vi "Digital Write Square Wave.vi"(7 "Duration (ms)":u32, 8 "Error In":errorcluster, 9 "Frequency":u16, 10 "DO Channel":u8, 11 "LINX Device Config":T1) -> (0 "Error Out":errorcluster, 3 "LINX Device Config":T1)   [LabVIEW 2013, in "LVH-LINX.lvlib" / "Device.lvlib"]
uses:
  <vilib>/LabVIEW Hacker/LINX/Private/Device/Device.lvlib
  <vilib>/LabVIEW Hacker/LINX/Private/Device/Type Defs/LINX Device Config.ctl
  <vilib>/LabVIEW Hacker/LINX/Private/Type Defs/Interface.ctl
  <vilib>/LabVIEW Hacker/LINX/Private/Device/Type Defs/TCP Config.ctl
  <vilib>/LabVIEW Hacker/LINX/Private/Type Defs/Device Family.ctl
  <vilib>/LabVIEW Hacker/LINX/Private/Type Defs/Error Type.ctl
  <vilib>/LabVIEW Hacker/LINX/LVH-LINX.lvlib
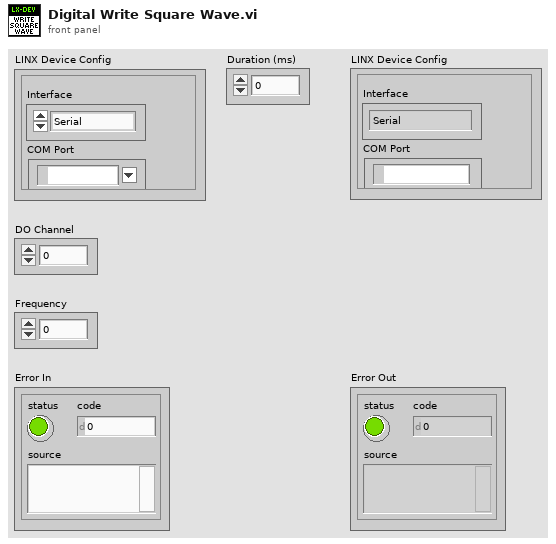
[diagram p1: front panel]
types:
  T1 = typedef "LVH-LINX.lvlib/Device.lvlib/LINX Device Config.ctl" = cluster{"Interface":T2, "COM Port":refnum<visa-resource-name>, "TCP Configuration":T3, "Device Family":T4, "Device ID":u8, "Device Name":string, "TCP Ref":refnum<k5>}
  T2 = typedef "LVH-LINX.lvlib/Interface.ctl" = enum16{"Serial", "TCP"}
  T3 = typedef "LVH-LINX.lvlib/Device.lvlib/TCP Config.ctl" = cluster{"IP Address":string, "Port":u16}
  T4 = typedef "LVH-LINX.lvlib/Device Family.ctl" = enum8{"National Instruments", "Digilent", "Arduino"}
  T5 = typedef "LVH-LINX.lvlib/Error Type.ctl" = enum16{"Unknown", "Timeout", "Corrupt Return Packet", "Unable To Connect", "Command Not Supported", "Channel DNE", "Invalid COM Config"}
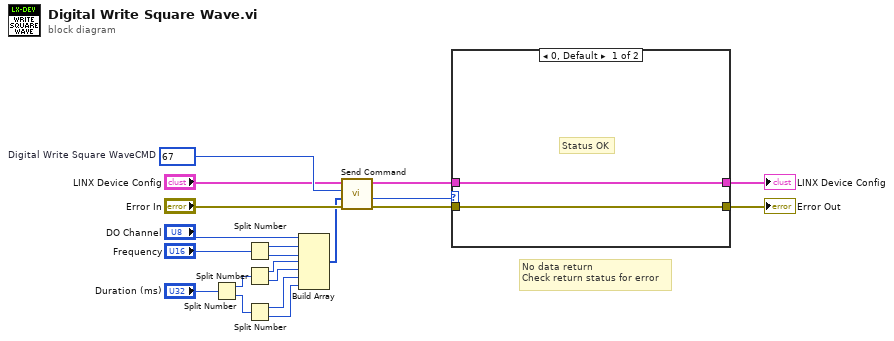
[diagram p0: block diagram]
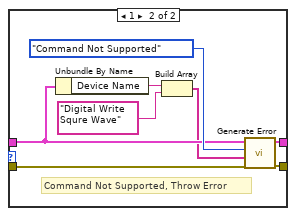
[diagram p2: hidden frame]
diagram:
  w19 = u16 67  # Digital Write Square WaveCMD
  # "No data return\nCheck return status for error"
  n1 = Split Number(x="Duration (ms)") -> (hi(x)=w5:u16, lo(x)=w6:u16)
  n2 = Split Number(x="Frequency") -> (hi(x)=w10:u8, lo(x)=w9:u8)
  n3 = Split Number(x=w5) -> (hi(x)=w4:u8, lo(x)=w3:u8)
  n4 = Split Number(x=w6) -> (hi(x)=w2:u8, lo(x)=w1:u8)
  n5 = Build Array("DO Channel", w10, w9, w4, w3, w2, w1) -> (w8:u8[])
  n6 = call <vilib>:"Send Command.vi"("Error In"="Error In", "ARGS"=w8, "CMD"=w19, "LINX Device Config"="LINX Device Config") -> ("Error Out"=w16:errorcluster, "Status"=w13:u8, "LINX Device Config"=w14:T1)  [unwired: 4 in, 1 out]
  n7 = case shown="0, Default" w13 {
    tunnel: [w22 w28] -> w18
    tunnel: w14 -> [w22 w24]
    tunnel: [w21 w29] -> w17
    tunnel: w16 -> [w21 w30]
    frame 0, Default {
      # "Status OK"
    }
    frame 1 {
      # "Command Not Supported, Throw Error"
      n8 = Unbundle By Name(w24) -> ("Device Name"=w26:string)
      n9 = Build Array(w26, "Digital Write Squre Wave") -> (w23:string[])
      n10 = call <vilib>:"Generate Error.vi"("Error In"=w30, "Arguments"=w23, "Error Type"=Error_Type."Command Not Supported", "LINX Device Config"=w24) -> ("Error Out"=w29:errorcluster, "LINX Device Config"=w28:T1)  [unwired: 6 in]
    }
  }
  "Error Out" <- w17
  "LINX Device Config" <- w18
